vi "zero_crossing.vi"(6 "Array in":dbl[](array[numeric]), 7 "Numeric 4":i32, 8 "Numeric in":dbl, 9 "zero detect down sampling rate in":i32, 10 "memory down sampling rate in":i32, 11 "Numeric 5":dbl) -> (0 "Waveform Graph 2":dbl[](graph), 1 "Array out":dbl[](array[numeric]), 2 "Numeric out":dbl, 3 "size(s) 2":i32, 4 "appended array 2":dbl[](array[numeric]), 5 "Numeric 3":i32)   [LabVIEW 2021]
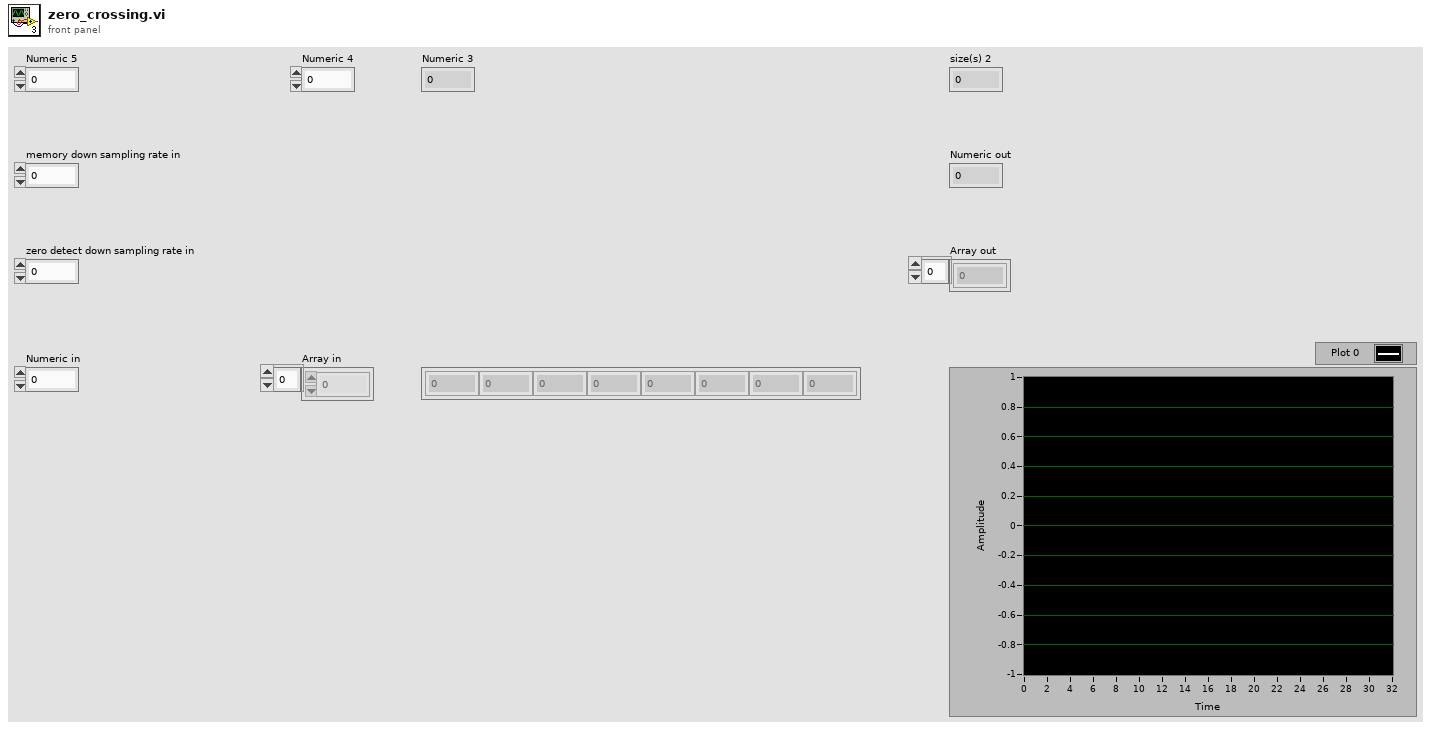
[diagram p1: front panel]
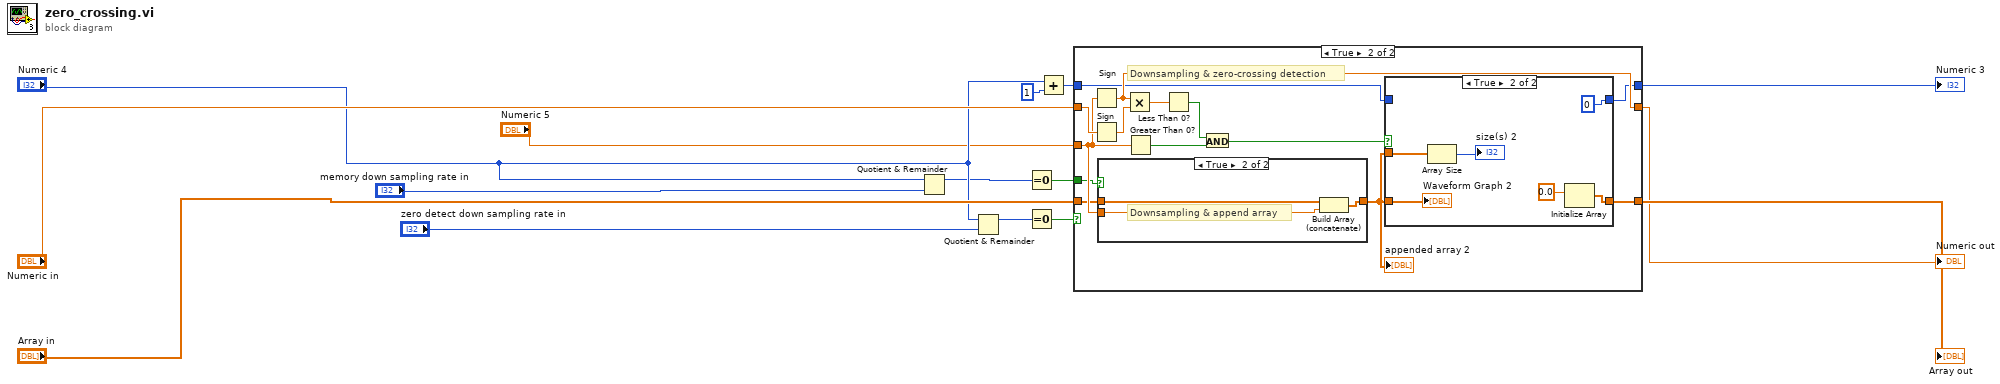
[diagram p0: block diagram]
diagram:
  n1 = Quotient & Remainder(x="Numeric 4", y="memory down sampling rate in") -> (x-y*floor(x/y)=w4:i32)  [unwired: 1 out]
  n2 = Quotient & Remainder(x="Numeric 4", y="zero detect down sampling rate in") -> (x-y*floor(x/y)=w1:i32)  [unwired: 1 out]
  n3 = Equal To 0?(x=w4) -> (x = 0?=w5:bool)
  n4 = Equal To 0?(x=w1) -> (x = 0?=w2:bool)
  n5 = Add(x="Numeric 4", y=1) -> (x+y=w7:i32)
  n6 = case shown="True" w2 {
    tunnel: "Numeric 5" -> [_ w27]
    tunnel: [w18 w30] -> w13
    tunnel: "Numeric in" -> [w18 w29]
    tunnel: [w17 w28] -> w15
    tunnel: "Array in" -> [w17 w21]
    tunnel: w5 -> [_ w19]
    tunnel: [w16 w23] -> w11
    tunnel: w7 -> [w16 w22]
    frame False {
    }
    frame True {
      # "Downsampling & zero-crossing detection"
      n7 = Sign(1:w27) -> (0:w30:dbl)
      n8 = Sign(1:w29) -> (0:w31:dbl)
      n9 = case shown="True" w19 {
        tunnel: w21 -> [w33 w36]
        tunnel: [w33 w35] -> w20
        tunnel: w27 -> [_ w34]
        frame False {
        }
        frame True {
          # "Downsampling & append array"
          n10 = Build Array (concatenate)(w36, w34) -> (w35:dbl[])
        }
      }
      "appended array 2" <- w20
      n11 = Multiply(x=w30, y=w31) -> (x*y=w32:dbl)
      n12 = Greater Than 0?(x=w27) -> (x > 0?=w25:bool)
      n13 = Less Than 0?(x=w32) -> (x < 0?=w26:bool)
      n14 = And(x=w26, y=w25) -> (x .and. y?=w24:bool)
      n15 = case shown="True" w24 {
        tunnel: w20 -> [w37 w40]
        tunnel: [w37 w44] -> w28
        tunnel: [w38 0] -> w23
        tunnel: w22 -> [w38 _]
        tunnel: w20 -> [_ w41]
        frame False {
        }
        frame True {
          n16 = Array Size(array=w41) -> (size(s)=→"size(s) 2":i32)
          n17 = Initialize Array(0.0 ("element")) -> (w44:dbl[])  [unwired: 1 in]
          "Waveform Graph 2" <- w40
        }
      }
    }
  }
  "Array out" <- w15
  "Numeric out" <- w13
  "Numeric 3" <- w11
